vi "TurnONRamp.vi"() -> ()   [LabVIEW 2013, in "ovenCtrl.lvlib"]
uses:
  ovenCtrl.lvlib
panel:
  out "Output Reading 3":string
  out "Output Reading 2":string
  out "Output Reading":string
  in  "error in (no error)":errorcluster
  out "error out":errorcluster
  in  "Port Number":u16=2000
  in  "IP Address":string="192.168.12.200"
  # "Inputs"
  # "Outputs"
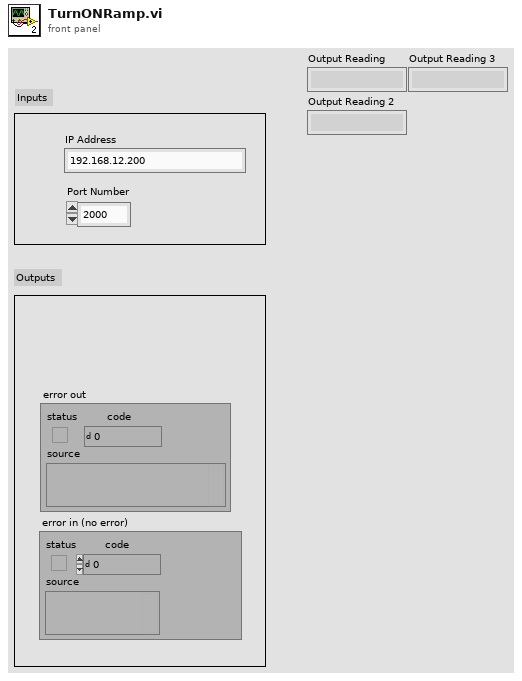
[diagram p1: front panel]
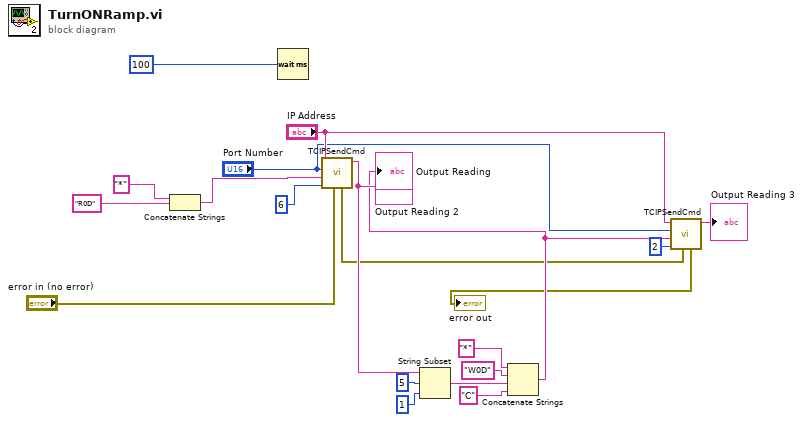
[diagram p0: block diagram]
diagram:
  n1 = Concatenate Strings("*" ("string"), "R0D" ("string")) -> (w17:string)
  n2 = Wait (ms)(milliseconds to wait=u32 100) -> ()  [unwired: 1 out]
  n3 = call "TCIPSendCmd.vi"("error in (no error)"="error in (no error)", "bytes to read"=6, "Command"=w17, "Port Number"="Port Number", "IP Address"="IP Address") -> ("Output Reading"=w11:string, "error out"=w3:errorcluster)  [unwired: 5 in]
  "Output Reading 2" <- w11
  n4 = String Subset(string=w11, offset (0)=5, length (rest)=1 ("length (rest)")) -> (substring=w9:string)
  n5 = Concatenate Strings("*" ("string"), "W0D" ("string"), w9, "C" ("string")) -> (w5:string)
  "Output Reading" <- w5
  n6 = call "TCIPSendCmd.vi"("error in (no error)"=w3, "bytes to read"=2, "Command"=w5, "Port Number"="Port Number", "IP Address"="IP Address") -> ("Output Reading"=→"Output Reading 3":string, "error out"=→"error out":errorcluster)  [unwired: 5 in]
